vi "Count Up U64.vi"(0 "increment":bool=TRUE, 1 "reset":bool) -> (4 "count out":u64)   [LabVIEW 2015, in "Engine Simulation Toolkit.lvlib"]
uses:
  Engine Simulation Toolkit.lvlib
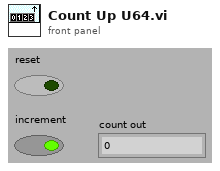
[diagram p1: front panel]
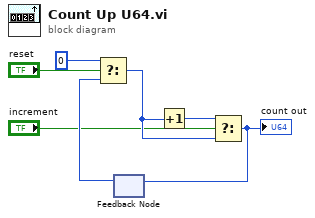
[diagram p0: block diagram]
diagram:
  n1 = feedback #1() -> (w5:u64)  [unwired: 1 in]
  n2 = Select(t=u64 0 ("count in"), s="reset", f=w5) -> (s? t:f=w6:u64)
  n3 = Increment(x=w6) -> (x+1=w7:u64)
  n4 = Select(t=w7, s="increment", f=w6) -> (s? t:f=w1:u64)
  "count out" <- w1
  n5 = feedback-in #1(w1) -> ()
